vi "Action Single Trigger.vi"(8 "error in (no error)":errorcluster, 11 "RS Z2X in":refnum<class "RS Z2X.lvclass">) -> (0 "error out":errorcluster, 3 "RS Z2X out":refnum<class "RS Z2X.lvclass">)   [LabVIEW 2020, in "RS Z2X.lvclass"]
uses:
  RS Z2X.lvclass
  C:/Sandbox/Git_Sandbox/WiSpry Test Framework source code (LV20)/WiSpry Test Framework/Instruments/Instrument.lvclass
  Instrument.lvclass/Instrument.ctl
  Instrument.lvclass
panel:
  out "Numeric":i32
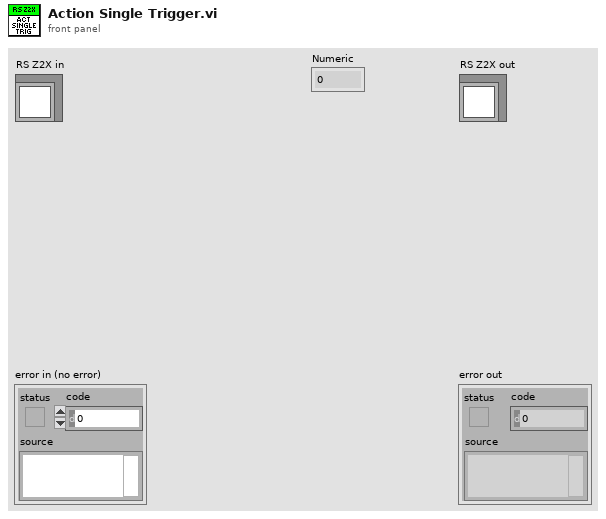
[diagram p1: front panel]
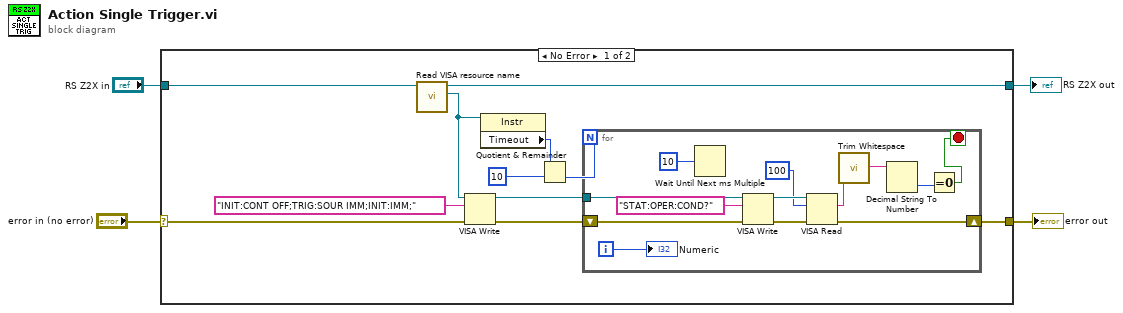
[diagram p0: block diagram]
diagram:
  n1 = case shown="No Error" "error in (no error)" {
    selector: "error in (no error)" -> [w13 w29]
    tunnel: "RS Z2X in" -> [w15 w30]
    tunnel: [w14 w30] -> w2
    tunnel: [w5 w29] -> w1
    frame No Error {
      n2 = call "Read VISA resource name.vi"("Instrument in"=w15) -> ("VISA resource name"=w11:refnum<visa-resource-name>, "Instrument out"=w14:refnum<class "RS Z2X.lvclass">)  [unwired: 9 in]
      n3 = VISA Write(VISA resource name=w11, write buffer="INIT:CONT OFF;TRIG:SOUR IMM;INIT:IMM;", error in (no error)=w13) -> (VISA resource name out=w6:refnum<visa-resource-name>, error out=w10:errorcluster)  [unwired: 1 out]
      n4 = property class="Instr"(reference=w11) -> ("Timeout"=w9:u32)  [unwired: 1 in, 2 out]
      n5 = Quotient & Remainder(x=w9, y=u32 10) -> (floor(x/y)=w7:u32)  [unwired: 1 out]
      n6 = for {
        N: w7 -> [_]
        shift-right: [w19] -> w5
        shift-left: w10 -> [w27]
        tunnel: w6 -> [w26]
        i -> [w16]
        stop <- w17 stop-if-true
        n7 = Wait Until Next ms Multiple(millisecond multiple=u32 10) -> ()  [unwired: 1 out]
        n8 = VISA Write(VISA resource name=w26, write buffer="STAT:OPER:COND?", error in (no error)=w27) -> (VISA resource name out=w23:refnum<visa-resource-name>, error out=w24:errorcluster)  [unwired: 1 out]
        n9 = VISA Read(VISA resource name=w23, byte count=u32 100, error in (no error)=w24) -> (read buffer=w21:string, error out=w19:errorcluster)  [unwired: 2 out]
        n10 = call <vilib>:"Trim Whitespace.vi"("string"=w21) -> ("trimmed string"=w20:string)  [unwired: 1 in]
        n11 = Decimal String To Number(string=w20) -> (number=w18:i32)  [unwired: 2 in, 1 out]
        n12 = Equal To 0?(x=w18) -> (x = 0?=w17:bool)
        "Numeric" <- w16
      }
    }
    frame Error {
    }
  }
  "error out" <- w1
  "RS Z2X out" <- w2
